vi "Actor Core.vi"(8 "error in":errorcluster, 11 "Test Executive Builder Active Path View In":refnum<class "Test Executive Builder Active Path View.lvclass">) -> (0 "error out":errorcluster, 3 "Actor out":refnum<class "Actor.lvclass">)   [LabVIEW 2017, in "Test Executive Builder Active Path View.lvclass"]
doc: "(<B>Filename</B>: Actor Framework.lvlib:Actor.lvclass:Actor Core.vi)\n\nReceives messages to the actor, reacts to them, and initiates any error handling that may shut the actor down.\n\nDescendant classes may override this VI to append parallel tasks for the actor to complete while it handles messages. Overrides use the Call Parent Method node.\n\n<License>\nCopyright © 2017 Composed Systems, LLC | All rights reserved\nwww.composed.io\n\nAuthor: Ethan Stern <ethan.stern@composed.io>\n\nThis software is provided \"AS IS\" WITHOUT WARRANTIES, either express or implied, AND IS FOR EDUCATIONAL PURPOSES ONLY.\n</License>"
uses:
  Test Executive Builder Active Path View.lvclass
  <vilib>/gpm_packages/@cs/mva-viewable/Source/IViewable/IViewable/IViewable.lvclass
  <vilib>/gpm_packages/@cs/mva-core/Source/IObserver/IObserver/IObserver.lvclass
  <vilib>/gpm_packages/@cs/mva-core/Source/SubscriptionPolicy/BasicSubscription/BasicSubscription.lvclass
  Test Executive Builder Active Path View Messages/Update Path Msg/Update Path Msg.lvclass
  C:/Users/jonmc/Documents/Git/Test Executive Builder/gpm_packages/@cs/mva-core/Source/IMediator/ISubscriptionPolicy/ISubscriptionPolicy.lvclass
  C:/Users/jonmc/Documents/Git/Test Executive Builder/gpm_packages/@cs/transport/Source/Concrete/ActorMessageTransport/Notification Msg/Notification Msg.lvclass
  C:/Users/jonmc/Documents/Git/Test Executive Builder/gpm_packages/@cs/mva-core/Source/IObserver/IObserver/IObserver.lvclass
  <vilib>/ActorFramework/Actor/Actor.lvclass
panel:
  out "Active Test Executive Path":string
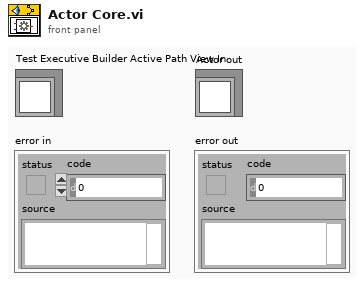
[diagram p1: front panel]
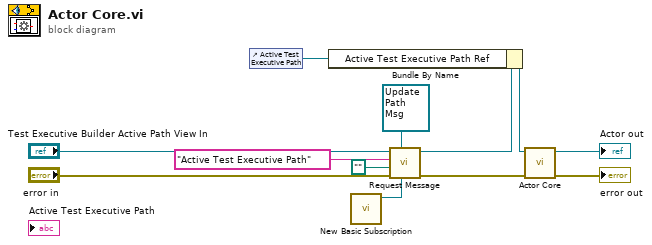
[diagram p0: block diagram]
diagram:
  n1 = control-ref of="Active Test Executive Path"() -> (w9:refnum<vi>)
  n2 = call <vilib>:"New Basic Subscription.vi"() -> ("BasicSubscription Out"=w8:refnum<class "BasicSubscription.lvclass">)  [unwired: 11 in]
  n3 = call <vilib>:"Request Message.vi"("Configured SubscriptionPolicy"=w8, "Desired Notification Msg"=refnum<class "Update Path Msg.lvclass"> refnum ("Update Path Msg.lvclass"), "error in (no error)"="error in", "Data Type"=path "", "Datum Name"="Active Test Executive Path", "IObserver in"="Test Executive Builder Active Path View In") -> ("error out"=w4:errorcluster, "IObserver out"=w6:refnum<class "Test Executive Builder Active Path View.lvclass">)  [unwired: 3 in, 1 out]
  n4 = Bundle By Name(cluster=w6, "Active Test Executive Path Ref"=w9) -> (w10:refnum<class "Test Executive Builder Active Path View.lvclass">)
  n5 = call-parent "Actor Core.vi"("error in"=w4, "IViewable In"=w10) -> ("error out"=→"error out":errorcluster, "Actor out"=→"Actor out":refnum<class "Actor.lvclass">)  [unwired: 8 in]
